vi "IOTest Host.vi"() -> ()   [LabVIEW 2012]
uses:
  <vilib>/FPGAPlugInAG/PCI-7831R/niLvFpga_Open_PCI-7831R.vi
  <vilib>/rvi/interface/common/dynamic/niFpgaDynamicAddResources.vi
  <vilib>/Utility/error.llb/Error Cluster From Error Code.vi
  <vilib>/rvi/errors/niLvFpgaAdjustHostInterfaceError.vi
  <vilib>/FPGAPlugInAG/Dynamic/niLvFpga_Close_Dynamic.vi
  <vilib>/rvi/interface/nirviOpenFPGA/nirviOpenFPGA.xnode
  SB130-XPS/Documents/FPGA-project-apporach-retraction/FPGA Bitfiles/Apporach-Retract_FPGATarget_IOTestTarget_tkpzxrrq7bY.lvbitx
  <vilib>/rvi/interface/nirviReadWriteControl/nirviReadWriteControl.xnode
  <vilib>/rvi/interface/nirviCloseFPGA/nirviCloseFPGA.xnode
  NiFpgaLv.dll
  <vilib>/rvi/interface/Simulation/niFpgaSimulationCallBeginRW.vi
panel:
  in  "Frequency":i32
  in  "Wait (ms)":i32
  out "Sine Signal":i16(graph)
  in  "Start":bool
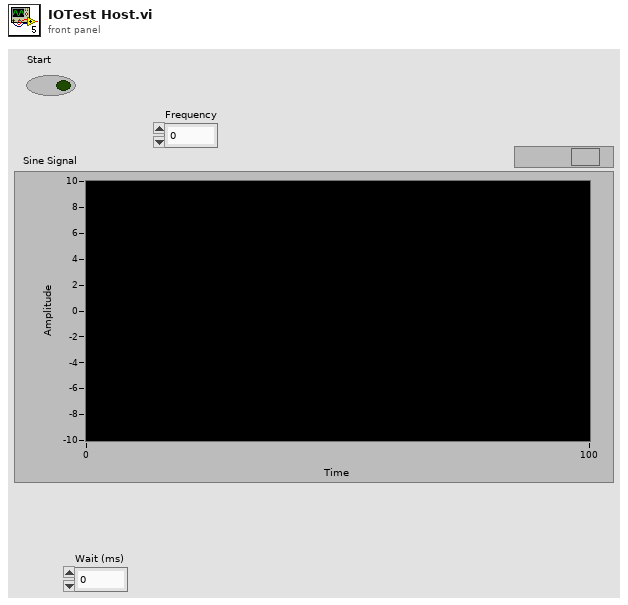
[diagram p1: front panel]
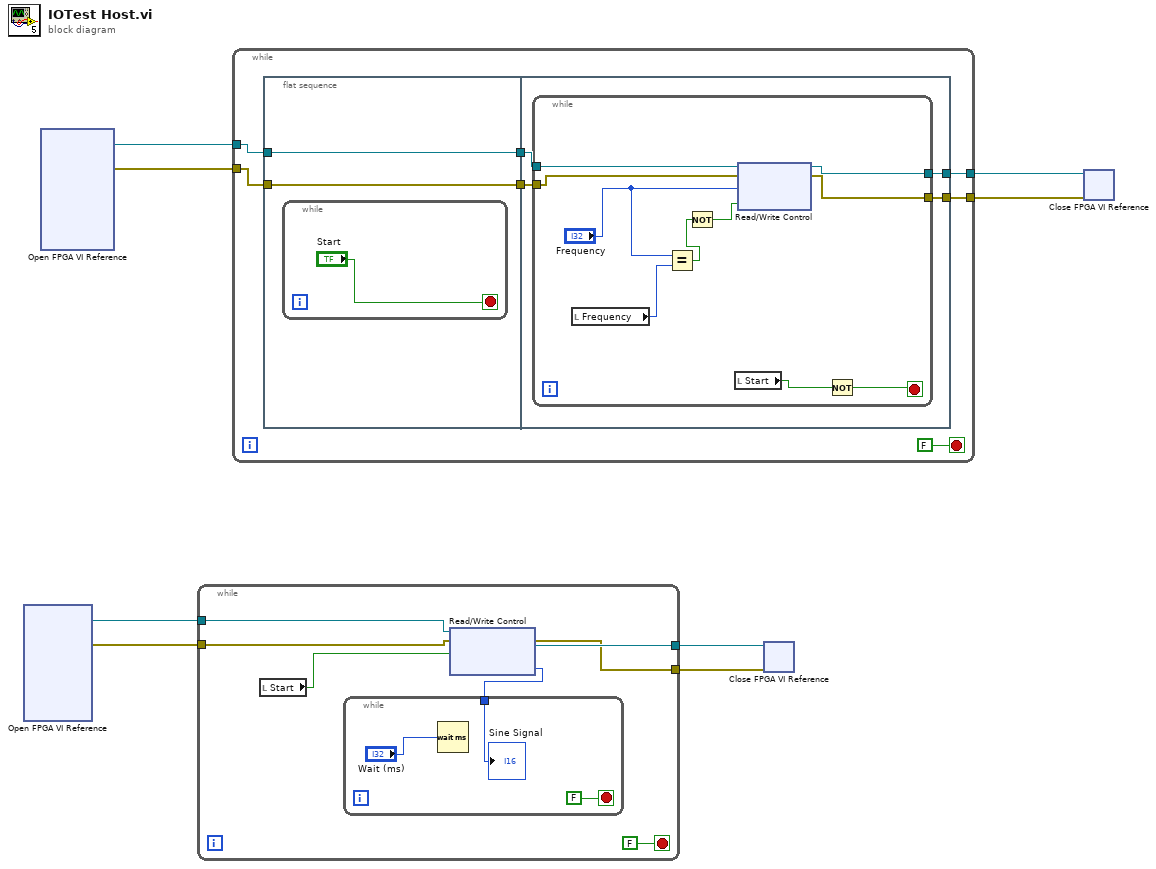
[diagram p0: block diagram]
diagram:
  n1 = xnode "Open FPGA VI Reference"() -> ("FPGA VI Reference Out"=w6:refnum<k20>, "error out"=w5:errorcluster)  [unwired: 2 in]
  n2 = xnode "Open FPGA VI Reference"() -> ("FPGA VI Reference Out"=w8:refnum<k20>, "error out"=w7:errorcluster)  [unwired: 2 in]
  n3 = while {
    tunnel: w6 -> [w14]
    tunnel: w5 -> [w13]
    tunnel: [w12] -> w4
    tunnel: [w11] -> w3
    stop <- FALSE stop-if-true
    n4 = local read "Start"() -> (w10:bool)
    n5 = xnode "Read/Write Control"("FPGA VI Reference In"=w14, "error in"=w13, "Start"=w10) -> ("FPGA VI Reference Out"=w12:refnum<k20>, "error out"=w11:errorcluster, "Signal Graph"=w9:i16)
    n6 = while {
      tunnel: w9 -> [w18]
      stop <- FALSE stop-if-true
      n7 = Wait (ms)(milliseconds to wait="Wait (ms)") -> ()  [unwired: 1 out]
      "Sine Signal" <- w18
    }
  }
  n8 = while {
    tunnel: w8 -> [w23]
    tunnel: w7 -> [w21]
    tunnel: [w20] -> w2
    tunnel: [w19] -> w1
    stop <- FALSE stop-if-true
    n9 = flat-sequence {
      tunnel: [w27] -> w24
      tunnel: w23 -> [w27]
      tunnel: [w26] -> w22
      tunnel: w21 -> [w26]
      tunnel: w24 -> [w32]
      tunnel: w22 -> [w31]
      tunnel: [w30] -> w20
      tunnel: [w29] -> w19
      frame #0 {
        n10 = while {
          stop <- "Start" stop-if-true
        }
      }
      frame #1 {
        n11 = while {
          tunnel: w32 -> [w40]
          tunnel: w31 -> [w39]
          tunnel: [w38] -> w30
          tunnel: [w37] -> w29
          stop <- w41 stop-if-true
          n12 = local read "Frequency"() -> (w36:i32)
          n13 = Equal?(x="Frequency", y=w36) -> (x = y?=w33:bool)
          n14 = Not(x=w33) -> (.not. x?=w34:bool)
          n15 = local read "Start"() -> (w42:bool)
          n16 = xnode "Read/Write Control"("FPGA VI Reference In"=w40, "error in"=w39, "Frequency"="Frequency", "Load"=w34) -> ("FPGA VI Reference Out"=w38:refnum<k20>, "error out"=w37:errorcluster)
          n17 = Not(x=w42) -> (.not. x?=w41:bool)
        }
      }
    }
  }
  n18 = xnode "Close FPGA VI Reference"("FPGA VI Reference In"=w4, "error in"=w3) -> ()  [unwired: 1 out]
  n19 = xnode "Close FPGA VI Reference"("FPGA VI Reference In"=w2, "error in"=w1) -> ()  [unwired: 1 out]
